vi "Configure Output Modulation.vi"(5 "External Modulation Type (0: Voltage Controlled Amplitude)":u16(ring) items=["Voltage Controlled Amplitude", "Suppressed Carrier Modulation"], 6 "Amplitude Modulation Depth (0 %)":dbl, 7 "Suppressed Carrier Modulation Level (0 V)":dbl, 8 "error in (no error)":errorcluster, 9 "Previous Channel Modulation Type (0: Amplitude Modulation)":u16(ring) items=["Amplitude Modulation", "Suppressed Carrier Modulation"], 10 "Output Modulation Source (1: Off)":u16(ring)=1 items=["External Modulation", "Off", "Previous Channel"], 11 "VISA resource name":refnum<visa-resource-name>) -> (0 "error out":errorcluster, 3 "VISA resource name out":refnum<visa-resource-name>)   [LabVIEW 2015, in "Fluke 28x Series.lvlib"]
doc: "Modulates output waveforms by amplitude. The modulation can be carried out by internal (another channel) or external means."
uses:
  <instrlib>/Fluke 28x Series/Fluke 28x Series.lvlib
panel:
  # "Previous Channel Output Modulation Source"
  # "External Output Modulation Source"
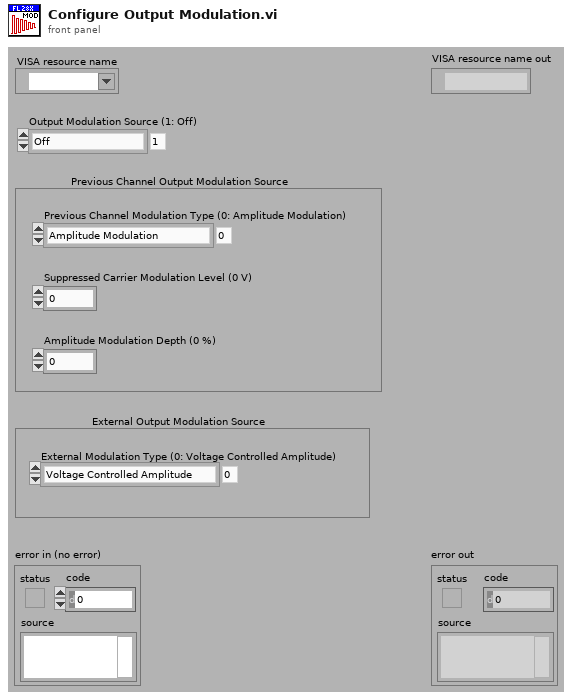
[diagram p1: front panel]
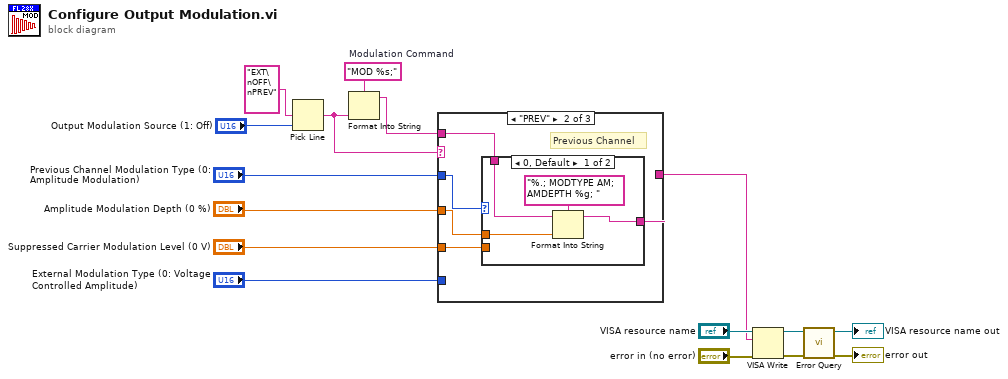
[diagram p0: block diagram]
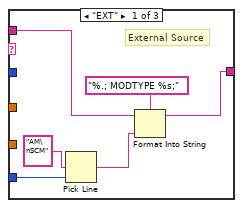
[diagram p2: hidden frame]
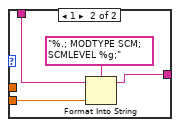
[diagram p3: hidden frame]
diagram:
  w12 = "MOD %s;"  # Modulation Command
  n1 = Pick Line(multi-line string="EXT\nOFF\nPREV", line index="Output Modulation Source (1: Off)") -> (output string=w5:string)  [unwired: 1 in]
  n2 = Format Into String(format string=w12, w5) -> (resulting string=w4:string)  [unwired: 2 in, 1 out]
  n3 = case shown="\"PREV\"" w5 {
    tunnel: "Amplitude Modulation Depth (0 %)" -> [_ w26 _]
    tunnel: "Suppressed Carrier Modulation Level (0 V)" -> [_ w24 _]
    tunnel: "Previous Channel Modulation Type (0: Amplitude Modulation)" -> [_ w27 _]
    tunnel: "External Modulation Type (0: Voltage Controlled Amplitude)" -> [w21 _ _]
    tunnel: [w19 w25 w36] -> w3
    tunnel: w4 -> [w18 w23 w36]
    frame "EXT" {
      # "External Source"
      n4 = Pick Line(multi-line string="AM\nSCM" ("string (\"\")"), line index=w21) -> (output string=w20:string)  [unwired: 1 in]
      n5 = Format Into String(format string="%.; MODTYPE %s;", initial string=w18, w20) -> (resulting string=w19:string)  [unwired: 1 in, 1 out]
    }
    frame "PREV" {
      # "Previous Channel"
      n6 = case shown="0, Default" w27 {
        tunnel: w26 -> [w30 _]
        tunnel: [w29 w35] -> w25
        tunnel: w24 -> [_ w34]
        tunnel: w23 -> [w28 w32]
        frame 0, Default {
          n7 = Format Into String(format string="%.; MODTYPE AM;  AMDEPTH %g; ", initial string=w28, w30) -> (resulting string=w29:string)  [unwired: 1 in, 1 out]
        }
        frame 1 {
          n8 = Format Into String(format string="%.; MODTYPE SCM; SCMLEVEL %g;", initial string=w32, w34) -> (resulting string=w35:string)  [unwired: 1 in, 1 out]
        }
      }
    }
    frame "OFF", Default {
      # "Modulation off"
    }
  }
  n9 = VISA Write(VISA resource name="VISA resource name", write buffer=w3, error in (no error)="error in (no error)") -> (VISA resource name out=w8:refnum<visa-resource-name>, error out=w7:errorcluster)  [unwired: 1 out]
  n10 = call <instrlib>:"Error Query.vi"("error in (no error)"=w7, "VISA resource name"=w8) -> ("error out"=→"error out":errorcluster, "VISA resource name out"=→"VISA resource name out":refnum<visa-resource-name>)  [unwired: 6 in, 2 out]
